vi "H5Tget_member_value.vi"   [LabVIEW 2017]
doc: "Returns the value of an enumeration datatype member.\n\n<p>"
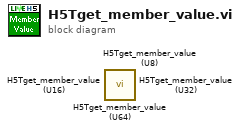
[diagram p0: block diagram]
diagram:
  n1 = call <vilib>:"H5Tget_member_value (U64).vi"() -> ()  [unwired: 7 in, 3 out]
  n2 = call <vilib>:"H5Tget_member_value (U8).vi"() -> ()  [unwired: 7 in, 3 out]
  n3 = call <vilib>:"H5Tget_member_value (U16).vi"() -> ()  [unwired: 7 in, 3 out]
  n4 = call <vilib>:"H5Tget_member_value (U32).vi"() -> ()  [unwired: 7 in, 3 out]
